vi "Emballage_BDD_insert_portcom.vi"(8 "entrée d'erreur (pas d'erreur)":errorcluster, 11 "portcom":string) -> (0 "sortie d'erreur":errorcluster)   [LabVIEW 2020]
uses:
  Modules/FS/60_FS_Controles/60_FS_SetGet.ctl
  <vilib>/drjdpowell/SQLite Library/SQL Connection/Open (path).vi
  <vilib>/drjdpowell/SQLite Library/SQL Connection/Open (string).vi
  <vilib>/AdvancedString/Path To Command Line String.vi
  <vilib>/drjdpowell/SQLite Library/SQL Connection/Connection.lvclass
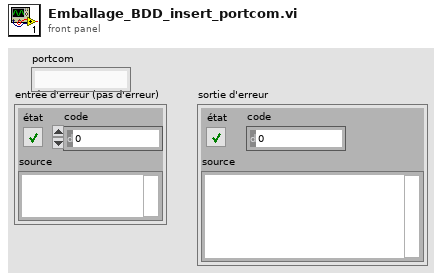
[diagram p1: front panel]
types:
  T1 = typedef "60_FS_SetGet.ctl" = enum16{"set", "get"}
  T2 = typedef "60_FS_CLT_Chemins.ctl" = cluster{"Racine_local":path, "Racine_reseau":path, "Racine_Support_Application":path, "Fichier_Journalisation":path, "Connexion_BDD_VSX":path, "Connexion_BDD_PLZ":path}
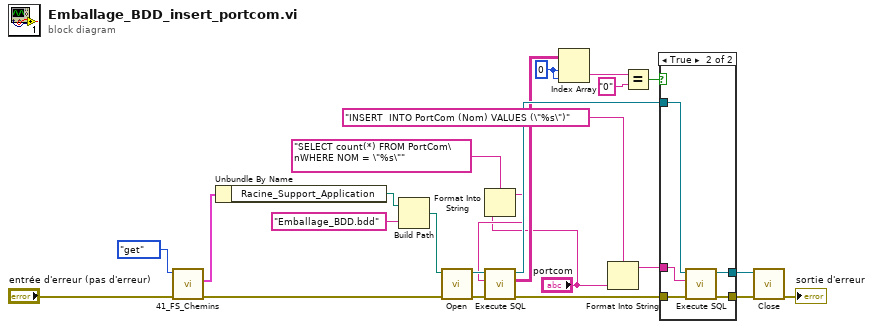
[diagram p0: block diagram]
diagram:
  w7 = 0 ("indice (ligne)")
  n1 = call "41_FS_Chemins.vi"("error in (no error)"="entrée d'erreur (pas d'erreur)", "SetGet"=60_FS_SetGet."get") -> ("error out"=w15:errorcluster, "CLT_Chemins_out"=w14:T2)  [unwired: 8 in]
  n2 = Unbundle By Name(w14) -> ("Racine_Support_Application"=w17:path)
  n3 = Build Path(base path=w17, name or relative path="Emballage_BDD.bdd" ("nom ou chemin relatif")) -> (appended path=w16:path)
  n4 = call-poly <vilib>:"Open.vi"("error in (no error)"=w15, "db file"=w16) -> ("error out"=w12:errorcluster, "SQLite Connection"=w10:refnum<class "Connection.lvclass">)  [unwired: 8 in]
  n5 = Format Into String(format string="SELECT count(*) FROM PortCom\nWHERE NOM = \"%s\"" ("SQL"), "portcom") -> (resulting string=w2:string)  [unwired: 2 in, 1 out]
  n6 = call <vilib>:"Execute SQL.vi"("error in (no error)"=w12, "SQL"=w2, "SQLite Connection in"=w10) -> ("error out"=w11:errorcluster, "Result Set"=w8:string[][], "SQLite Connection"=w9:refnum<class "Connection.lvclass">)  [unwired: 5 in, 1 out]
  n7 = Index Array(array=w8, index (row)=w7, index (col)=w7) -> (element=w6:string)
  n8 = Format Into String(format string="INSERT  INTO PortCom (Nom) VALUES (\"%s\")" ("SQL"), "portcom") -> (resulting string=w13:string)  [unwired: 2 in, 1 out]
  n9 = Equal?(x=w6, y="0") -> (x = y?=w4:bool)
  n10 = case shown="True" w4 {
    tunnel: [w26 w31] -> w19
    tunnel: [w25 w30] -> w18
    tunnel: w13 -> [_ w29]
    tunnel: w11 -> [w25 w28]
    tunnel: w9 -> [w26 w27]
    frame False {
    }
    frame True {
      n11 = call <vilib>:"Execute SQL.vi"("error in (no error)"=w28, "SQL"=w29, "SQLite Connection in"=w27) -> ("error out"=w30:errorcluster, "SQLite Connection"=w31:refnum<class "Connection.lvclass">)  [unwired: 5 in, 2 out]
    }
  }
  n12 = call-dynamic "Close.vi"("error in (no error)"=w18, "SQLite Connection in"=w19) -> ("error out"=→"sortie d'erreur":errorcluster)  [unwired: 9 in]
